vi "Set Caster Wheel Parameters.vi"(8 "error in (no error)":errorcluster, 10 "caster parameters":T1={"forward offset"=0.0, "caster gear ratio"=1.0}, 11 "caster wheel in":refnum<class "NI_Robotics_Caster Wheel.lvclass">) -> (0 "error out":errorcluster, 3 "caster wheel out":refnum<class "NI_Robotics_Caster Wheel.lvclass">)   [LabVIEW 2017, in "NI_Robotics_Caster Wheel.lvclass"]
uses:
  <vilib>/robotics/Steering/Caster Wheel/NI_Robotics_Caster Wheel.lvclass
  <vilib>/robotics/Steering/Caster Wheel/Caster Wheel Parameters.ctl
  <vilib>/robotics/Steering/Caster Wheel/NI_Robotics_Caster Wheel.lvclass/NI_Robotics_Caster Wheel.ctl
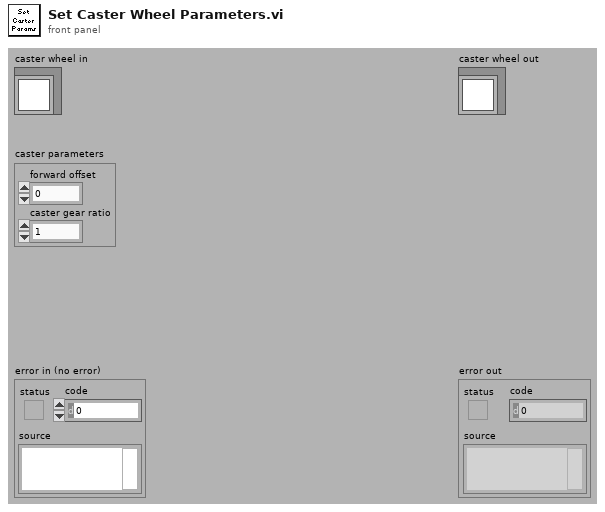
[diagram p1: front panel]
types:
  T1 = typedef "NI_Robotics_Caster Wheel.lvclass/Caster Wheel Parameters.ctl" = cluster{"forward offset":dbl, "caster gear ratio":dbl}
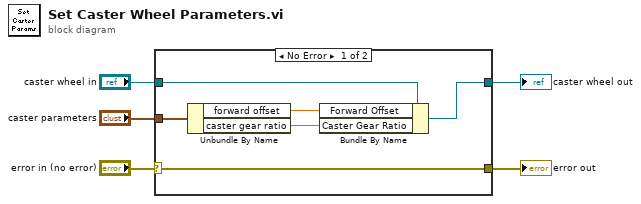
[diagram p0: block diagram]
diagram:
  n1 = case shown="No Error" "error in (no error)" {
    selector: "error in (no error)" -> [w11 w13]
    tunnel: [w11 w13] -> w4
    tunnel: [w6 w12] -> w2
    tunnel: "caster wheel in" -> [w7 w12]
    tunnel: "caster parameters" -> [w10 _]
    frame No Error {
      n2 = Unbundle By Name(w10) -> ("forward offset"=w9:dbl, "caster gear ratio"=w8:dbl)
      n3 = Bundle By Name(cluster=w7, "Forward Offset"=w9, "Caster Gear Ratio"=w8) -> (w6:refnum<class "NI_Robotics_Caster Wheel.lvclass">)
    }
    frame Error {
    }
  }
  "error out" <- w4
  "caster wheel out" <- w2
